vi "Request_int_JSON.vi"(0 "reference in":T1, 5 "method":string, 7 "params":variant, 9 "id":i32, 11 "error in (no error)":errorcluster) -> (4 "reference out":T1, 6 "response":variant, 15 "error out":errorcluster)   [LabVIEW 2017, in "JSON_RPC_client.lvlib"]
uses:
  JSON_RPC_client.lvlib
  reference.ctl
  <vilib>/httpClient/ClientHandle.ctl
  <vilib>/LVH/i3 JSON/JSON Generation/Create Value Files/Create Value - Object.vi
  <vilib>/LVH/i3 JSON/JSON Generation/Add Object Parameter Files/Add Object Parameter - String.vi
  <vilib>/LVH/i3 JSON/JSON Generation/Add Object Parameter Files/Add Object Parameter - Object.vi
  <vilib>/LVH/i3 JSON/JSON Generation/Add Object Parameter Files/Add Object Parameter - Numeric.vi
  <vilib>/httpClient/POSTBuffer.vi
  <vilib>/httpClient/LabVIEWHTTPClient.lvlib
  <vilib>/LVH/i3 JSON/i3-json.lvlib
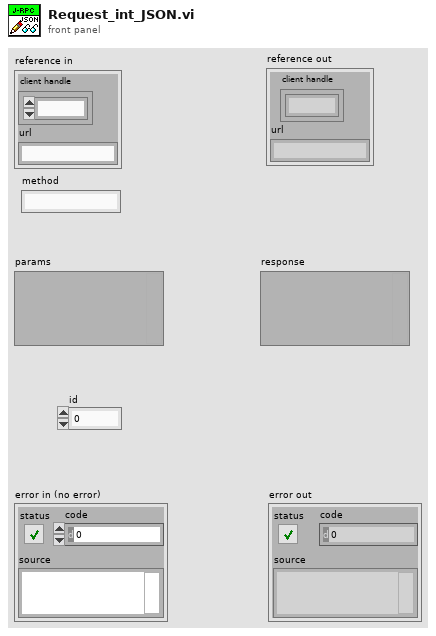
[diagram p1: front panel]
types:
  T1 = typedef "JSON_RPC_client.lvlib/reference.ctl" = cluster{"client handle":T2, "url":string}
  T2 = typedef "LabVIEWHTTPClient.lvlib/ClientHandle.ctl" = refnum<k1>
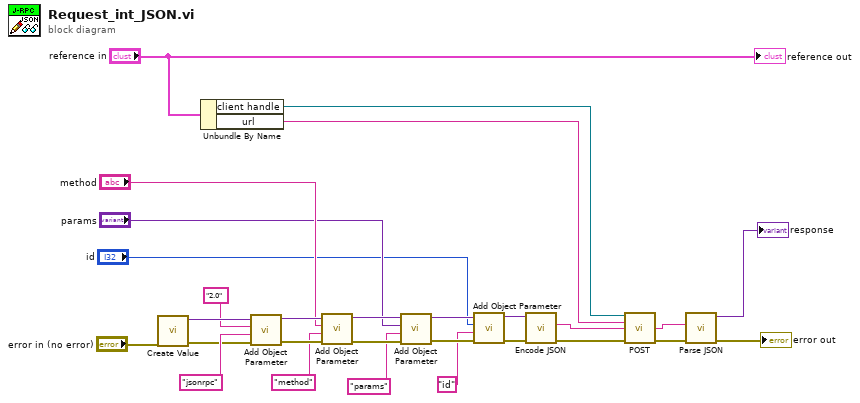
[diagram p0: block diagram]
diagram:
  n1 = call-poly <vilib>:"Create Value.vi"("error in (no error)"="error in (no error)") -> ("error out"=w21:errorcluster, "JSON Tree"=w25:variant)  [unwired: 9 in]
  n2 = Unbundle By Name("reference in") -> ("client handle"=w27:T2, "url"=w26:string)
  n3 = call-poly <vilib>:"Add Object Parameter.vi"("error in (no error)"=w21, "Name"="jsonrpc", "String"="2.0", "JSON Tree in (JSON Object)"=w25) -> ("error out"=w19:errorcluster, "JSON Tree out (JSON Object)"=w20:variant)  [unwired: 6 in]
  n4 = call-poly <vilib>:"Add Object Parameter.vi"("error in (no error)"=w19, "Name"="method", "String"="method", "JSON Tree in (JSON Object)"=w20) -> ("error out"=w15:errorcluster, "JSON Tree out (JSON Object)"=w16:variant)  [unwired: 6 in]
  n5 = call-poly <vilib>:"Add Object Parameter.vi"("error in (no error)"=w15, "Name"="params", "JSON Object"="params", "JSON Tree in (JSON Object)"=w16) -> ("error out"=w11:errorcluster, "JSON Tree out (JSON Object)"=w12:variant)  [unwired: 6 in]
  n6 = call-poly <vilib>:"Add Object Parameter.vi"("error in (no error)"=w11, "Name"="id", "Numeric"="id", "JSON Tree in (JSON Object)"=w12) -> ("error out"=w8:errorcluster, "JSON Tree out (JSON Object)"=w7:variant)  [unwired: 6 in]
  n7 = call <vilib>:"Encode JSON.vi"("error in (no error)"=w8, "JSON Tree"=w7) -> ("error out"=w5:errorcluster, "String"=w6:string)  [unwired: 4 in]
  n8 = call-poly <vilib>:"POST.vi"("client handle"=w27, "url"=w26, "buffer"=w6, "error in (no error)"=w5) -> ("body"=w3:string, "error out"=w4:errorcluster)  [unwired: 8 in, 2 out]
  n9 = call <vilib>:"Parse JSON.vi"("error in (no error)"=w4, "JSON String"=w3) -> ("error out"=→"error out":errorcluster, "JSON Tree"=→"response":variant)  [unwired: 6 in, 2 out]
  "reference out" <- "reference in"
